vi "Clone.vi"(0 "object in":refnum<class "Scripting.lvclass">, 5 "error in (no error)":errorcluster) -> (14 "object out":refnum<class "Scripting.lvclass">, 19 "error out":errorcluster)   [LabVIEW 2014, in "Scripting.lvclass"]
uses:
  <resource>/Framework/Providers/Open_GDS/ClassProviders/Common/ScriptingFunctions/Scripting.lvclass
  <resource>/Framework/Providers/Open_GDS/ClassProviders/Common/ScriptingFunctions/Scripting.lvclass/Scripting.ctl
panel:
  out "Cloned object out":refnum<class "Scripting.lvclass">
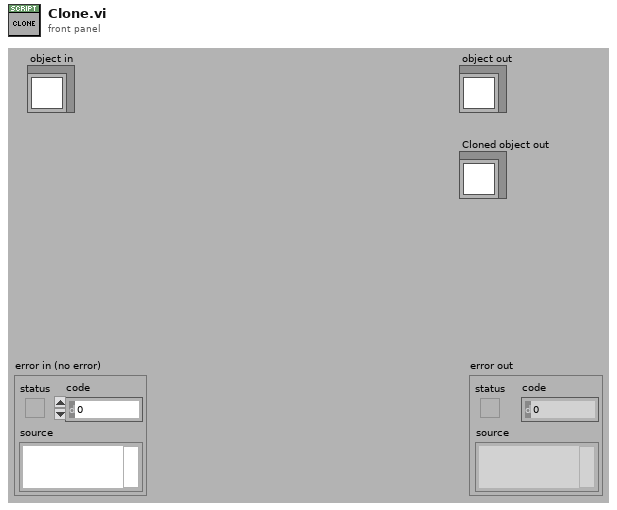
[diagram p1: front panel]
types:
  T1 = typedef "Scripting.lvclass/Scripting_PastThroughObjectType.ctl" = cluster{"Object":refnum<vi>, "InsideArray":bool, "PastThroughObjectTypes":T2[], "ObjectType":string, "ObjectData":string}
  T2 = typedef "Scripting_ObjectType.ctl" = cluster{"ObjectType":string, "ObjectName":string, "ObjectTerminalName":string}
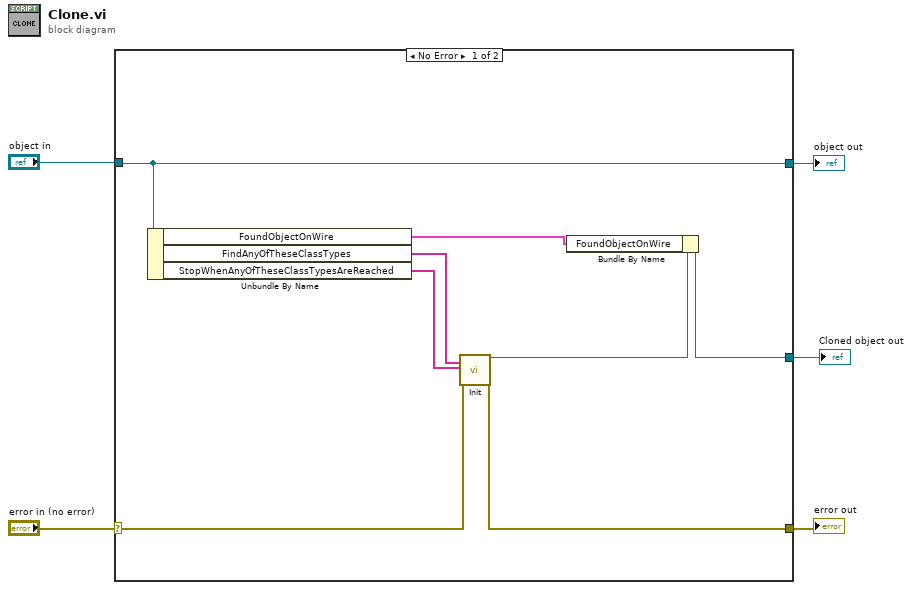
[diagram p0: block diagram]
diagram:
  n1 = case shown="No Error" "error in (no error)" {
    selector: "error in (no error)" -> [w7 w15]
    tunnel: [w6 w15] -> w4
    tunnel: [w11 w14] -> w2
    tunnel: "object in" -> [w11 w14]
    tunnel: [w8 _] -> w1
    frame No Error {
      n2 = Unbundle By Name(w11) -> ("FoundObjectOnWire"=w10:T1, "FindAnyOfTheseClassTypes"=w13:string[], "StopWhenAnyOfTheseClassTypesAreReached"=w12:string[])
      n3 = call <resource>:"Init.vi"("FindAnyOfTheseClassTypes"=w13, "StopWhenAnyOfTheseClassTypesAreReached"=w12, "error in (no error)"=w7) -> ("object out"=w9:refnum<class "Scripting.lvclass">, "error out"=w6:errorcluster)  [unwired: 15 in]
      n4 = Bundle By Name(cluster=w9, "FoundObjectOnWire"=w10) -> (w8:refnum<class "Scripting.lvclass">)
    }
    frame Error {
    }
  }
  "error out" <- w4
  "object out" <- w2
  "Cloned object out" <- w1
